vi "NM GlobalTest.vi"() -> ()   [LabVIEW 2010] (continued)
                            tunnel: w1850 -> [w1856 w1873]
                            tunnel: [w1856 w1871] -> w1849
                            tunnel: "data 13" -> [w1860 w1869]
                            tunnel: w1847 -> [w1859 w1868]
                            tunnel: w1846 -> [w1858 w1867]
                            tunnel: [w1857 w1866] -> w1845
                            frame "ULx", Default {
                              n548 = call-poly <vilib>:"ULx Write.vi"("task in"=w1864, "auto start"=w1858, "data"=w1860, "timeout"=w1859, "error in"=w1863) -> ("task out"=w1861:refnum<k24>, "number of samples written per channel"=w1857:u32, "error out"=w1862:errorcluster)  [unwired: 8 in]
                            }
                            frame "DAQmx" {
                              n549 = call-poly <vilib>:"DAQmx Write.vi"("task/channels in"=w1873, "auto start"=w1867, "data"=w1869, "timeout"=w1868, "error in"=w1872) -> ("task out"=w1871:refnum<k21>, "number of samples written per channel"=w1866:u32, "error out"=w1870:errorcluster)  [unwired: 8 in]
                            }
                          }
                        }
                        frame "nCsSU8" {
                          n550 = case shown="\"ULx\", Default" w1882 {
                            tunnel: [w1890 w1894] -> w1884
                            tunnel: [w1891 w1900] -> w1883
                            tunnel: w1881 -> [w1892 w1901]
                            tunnel: w1880 -> [w1893 w1894]
                            tunnel: [w1885 w1899] -> w1879
                            tunnel: w1878 -> [w1885 w1902]
                            tunnel: "data 14" -> [w1889 w1898]
                            tunnel: w1876 -> [w1888 w1897]
                            tunnel: w1875 -> [w1887 w1896]
                            tunnel: [w1886 w1895] -> w1874
                            frame "ULx", Default {
                              n551 = call-poly <vilib>:"ULx Write.vi"("task in"=w1893, "auto start"=w1887, "data"=w1889, "timeout"=w1888, "error in"=w1892) -> ("task out"=w1890:refnum<k24>, "number of samples written per channel"=w1886:u32, "error out"=w1891:errorcluster)  [unwired: 8 in]
                            }
                            frame "DAQmx" {
                              n552 = call-poly <vilib>:"DAQmx Write.vi"("task/channels in"=w1902, "auto start"=w1896, "data"=w1898, "timeout"=w1897, "error in"=w1901) -> ("task out"=w1899:refnum<k21>, "number of samples written per channel"=w1895:u32, "error out"=w1900:errorcluster)  [unwired: 8 in]
                            }
                          }
                        }
                        frame "nCsSU16" {
                          n553 = case shown="\"ULx\", Default" w1911 {
                            tunnel: [w1919 w1929] -> w1913
                            tunnel: [w1921 w1923] -> w1912
                            tunnel: w1910 -> [w1920 w1930]
                            tunnel: w1909 -> [w1922 w1923]
                            tunnel: [w1914 w1928] -> w1908
                            tunnel: w1907 -> [w1914 w1931]
                            tunnel: "data 15" -> [w1918 w1927]
                            tunnel: w1905 -> [w1917 w1925]
                            tunnel: w1904 -> [w1916 w1926]
                            tunnel: [w1915 w1924] -> w1903
                            frame "ULx", Default {
                              n554 = call-poly <vilib>:"ULx Write.vi"("task in"=w1922, "auto start"=w1916, "data"=w1918, "timeout"=w1917, "error in"=w1920) -> ("task out"=w1921:refnum<k24>, "number of samples written per channel"=w1915:u32, "error out"=w1919:errorcluster)  [unwired: 8 in]
                            }
                            frame "DAQmx" {
                              n555 = call-poly <vilib>:"DAQmx Write.vi"("task/channels in"=w1931, "auto start"=w1926, "data"=w1927, "timeout"=w1925, "error in"=w1930) -> ("task out"=w1928:refnum<k21>, "number of samples written per channel"=w1924:u32, "error out"=w1929:errorcluster)  [unwired: 8 in]
                            }
                          }
                        }
                        frame "nCsSU32" {
                          n556 = case shown="\"ULx\", Default" w1939 {
                            tunnel: [w1948 w1952] -> w1942
                            tunnel: [w1949 w1958] -> w1941
                            tunnel: w1940 -> [w1950 w1957]
                            tunnel: w1938 -> [w1951 w1952]
                            tunnel: [w1943 w1959] -> w1937
                            tunnel: w1936 -> [w1943 w1960]
                            tunnel: "data 16" -> [w1947 w1956]
                            tunnel: w1934 -> [w1946 w1955]
                            tunnel: w1933 -> [w1945 w1954]
                            tunnel: [w1944 w1953] -> w1932
                            frame "ULx", Default {
                              n557 = call-poly <vilib>:"ULx Write.vi"("task in"=w1951, "auto start"=w1945, "data"=w1947, "timeout"=w1946, "error in"=w1950) -> ("task out"=w1948:refnum<k24>, "number of samples written per channel"=w1944:u32, "error out"=w1949:errorcluster)  [unwired: 8 in]
                            }
                            frame "DAQmx" {
                              n558 = call-poly <vilib>:"DAQmx Write.vi"("task/channels in"=w1960, "auto start"=w1954, "data"=w1956, "timeout"=w1955, "error in"=w1957) -> ("task out"=w1959:refnum<k21>, "number of samples written per channel"=w1953:u32, "error out"=w1958:errorcluster)  [unwired: 8 in]
                            }
                          }
                        }
                        frame "nCsSWv" {
                          n559 = case shown="\"ULx\", Default" w1969 {
                            tunnel: [w1977 w1981] -> w1971
                            tunnel: [w1978 w1986] -> w1970
                            tunnel: w1968 -> [w1979 w1987]
                            tunnel: w1967 -> [w1980 w1981]
                            tunnel: w1966 -> [w1972 w1989]
                            tunnel: [w1972 w1988] -> w1965
                            tunnel: "data 17" -> [w1976 w1985]
                            tunnel: w1963 -> [w1975 w1984]
                            tunnel: [w1974 w1982] -> w1962
                            tunnel: w1961 -> [w1973 w1983]
                            frame "ULx", Default {
                              n560 = call-poly <vilib>:"ULx Write.vi"("task in"=w1980, "auto start"=w1973, "data"=w1976, "timeout"=w1975, "error in"=w1979) -> ("task out"=w1977:refnum<k24>, "number of samples written per channel"=w1974:u32, "error out"=w1978:errorcluster)  [unwired: 8 in]
                            }
                            frame "DAQmx" {
                              n561 = call-poly <vilib>:"DAQmx Write.vi"("task/channels in"=w1989, "auto start"=w1983, "data"=w1985, "timeout"=w1984, "error in"=w1987) -> ("task out"=w1988:refnum<k21>, "number of samples written per channel"=w1982:u32, "error out"=w1986:errorcluster)  [unwired: 8 in]
                            }
                          }
                        }
                        frame "nCnSU8" {
                          n562 = case shown="\"ULx\", Default" w1998 {
                            tunnel: [w2008 w2010] -> w2000
                            tunnel: [w2007 w2016] -> w1999
                            tunnel: w1997 -> [w2006 w2017]
                            tunnel: w1996 -> [w2009 w2010]
                            tunnel: w1995 -> [w2001 w2018]
                            tunnel: [w2001 w2015] -> w1994
                            tunnel: "data 18" -> [w2005 w2014]
                            tunnel: w1992 -> [w2004 w2013]
                            tunnel: w1991 -> [w2003 w2012]
                            tunnel: [w2002 w2011] -> w1990
                            frame "ULx", Default {
                              n563 = call-poly <vilib>:"ULx Write.vi"("task in"=w2009, "auto start"=w2003, "data"=w2005, "timeout"=w2004, "error in"=w2006) -> ("task out"=w2008:refnum<k24>, "number of samples written per channel"=w2002:u32, "error out"=w2007:errorcluster)  [unwired: 8 in]
                            }
                            frame "DAQmx" {
                              n564 = call-poly <vilib>:"DAQmx Write.vi"("task/channels in"=w2018, "auto start"=w2012, "data"=w2014, "timeout"=w2013, "error in"=w2017) -> ("task out"=w2015:refnum<k21>, "number of samples written per channel"=w2011:u32, "error out"=w2016:errorcluster)  [unwired: 8 in]
                            }
                          }
                        }
                        frame "nCnSU16" {
                          n565 = case shown="\"ULx\", Default" w2027 {
                            tunnel: [w2036 w2044] -> w2029
                            tunnel: [w2035 w2039] -> w2028
                            tunnel: w2026 -> [w2037 w2045]
                            tunnel: w2025 -> [w2038 w2039]
                            tunnel: [w2030 w2046] -> w2024
                            tunnel: w2023 -> [w2030 w2047]
                            tunnel: "data 19" -> [w2034 w2043]
                            tunnel: w2021 -> [w2033 w2042]
                            tunnel: w2020 -> [w2032 w2041]
                            tunnel: [w2031 w2040] -> w2019
                            frame "ULx", Default {
                              n566 = call-poly <vilib>:"ULx Write.vi"("task in"=w2038, "auto start"=w2032, "data"=w2034, "timeout"=w2033, "error in"=w2037) -> ("task out"=w2035:refnum<k24>, "number of samples written per channel"=w2031:u32, "error out"=w2036:errorcluster)  [unwired: 8 in]
                            }
                            frame "DAQmx" {
                              n567 = call-poly <vilib>:"DAQmx Write.vi"("task/channels in"=w2047, "auto start"=w2041, "data"=w2043, "timeout"=w2042, "error in"=w2045) -> ("task out"=w2046:refnum<k21>, "number of samples written per channel"=w2040:u32, "error out"=w2044:errorcluster)  [unwired: 8 in]
                            }
                          }
                        }
                        frame "nCnSU32" {
                          n568 = case shown="\"ULx\", Default" w2056 {
                            tunnel: [w2066 w2068] -> w2058
                            tunnel: [w2065 w2075] -> w2057
                            tunnel: w2055 -> [w2067 w2068]
                            tunnel: w2054 -> [w2064 w2074]
                            tunnel: [w2059 w2076] -> w2053
                            tunnel: w2052 -> [w2059 w2073]
                            tunnel: "data 20" -> [w2063 w2072]
                            tunnel: w2050 -> [w2062 w2071]
                            tunnel: w2049 -> [w2061 w2070]
                            tunnel: [w2060 w2069] -> w2048
                            frame "ULx", Default {
                              n569 = call-poly <vilib>:"ULx Write.vi"("task in"=w2067, "auto start"=w2061, "data"=w2063, "timeout"=w2062, "error in"=w2064) -> ("task out"=w2066:refnum<k24>, "number of samples written per channel"=w2060:u32, "error out"=w2065:errorcluster)  [unwired: 8 in]
                            }
                            frame "DAQmx" {
                              n570 = call-poly <vilib>:"DAQmx Write.vi"("task/channels in"=w2073, "auto start"=w2070, "data"=w2072, "timeout"=w2071, "error in"=w2074) -> ("task out"=w2076:refnum<k21>, "number of samples written per channel"=w2069:u32, "error out"=w2075:errorcluster)  [unwired: 8 in]
                            }
                          }
                        }
                        frame "nCnSWv" {
                          n571 = case shown="\"ULx\", Default" w2085 {
                            tunnel: [w2096 w2105] -> w2087
                            tunnel: [w2095 w2097] -> w2086
                            tunnel: w2084 -> [w2094 w2097]
                            tunnel: w2083 -> [w2088 w2104]
                            tunnel: w2082 -> [w2093 w2103]
                            tunnel: [w2088 w2102] -> w2081
                            tunnel: "data 21" -> [w2092 w2101]
                            tunnel: w2079 -> [w2091 w2100]
                            tunnel: w2078 -> [w2090 w2099]
                            tunnel: [w2089 w2098] -> w2077
                            frame "ULx", Default {
                              n572 = call-poly <vilib>:"ULx Write.vi"("task in"=w2094, "auto start"=w2090, "data"=w2092, "timeout"=w2091, "error in"=w2093) -> ("task out"=w2095:refnum<k24>, "number of samples written per channel"=w2089:u32, "error out"=w2096:errorcluster)  [unwired: 8 in]
                            }
                            frame "DAQmx" {
                              n573 = call-poly <vilib>:"DAQmx Write.vi"("task/channels in"=w2104, "auto start"=w2099, "data"=w2101, "timeout"=w2100, "error in"=w2103) -> ("task out"=w2102:refnum<k21>, "number of samples written per channel"=w2098:u32, "error out"=w2105:errorcluster)  [unwired: 8 in]
                            }
                          }
                        }
                      }
                    }
                    frame "Single Channel" {
                      n574 = call "AtoDSigConvert.vi"("Samples"=w2108, "Array Input"=w2109) -> ("sCnSu32"=w2106:u32[], "sCnSu16"=w2107:u16[], "sCnSu8"=w2110:u8[])
                      n575 = case shown="\"sCnSU32\"" "sDWrite" {
                        tunnel: [w2131 w2161 w2189 w2219 w2247 w2276 w2305 w2335 w2363 w2393] -> w2114
                        tunnel: [w2132 w2160 w2190 w2218 w2248 w2277 w2306 w2334 w2364 w2392] -> w2115
                        tunnel: w2117 -> [w2130 w2158 w2188 w2217 w2245 w2275 w2304 w2333 w2362 w2391]
                        tunnel: w2119 -> [w2128 w2159 w2186 w2215 w2244 w2273 w2302 w2331 w2361 w2390]
                        tunnel: w2120 -> [w2129 w2156 w2184 w2213 w2242 w2272 w2301 w2329 w2358 w2389]
                        tunnel: w2118 -> [w2127 w2157 w2187 w2216 w2246 w2274 w2303 w2332 w2360 w2388]
                        tunnel: [w2126 w2155 w2185 w2214 w2243 w2271 w2300 w2330 w2359 w2387] -> w2116
                        tunnel: w2113 -> [w2123 w2153 w2181 w2210 w2239 w2269 w2298 w2327 w2356 w2384]
                        tunnel: w2112 -> [w2124 w2152 w2182 w2211 w2240 w2267 w2299 w2328 w2357 w2385]
                        tunnel: [w2122 w2151 w2180 w2209 w2238 w2268 w2297 w2326 w2355 w2383] -> w2111
                        tunnel: w2110 -> [_ _ _ _ _ _ w2296 _ _ _]
                        tunnel: w2107 -> [_ _ _ _ _ _ _ w2325 _ _]
                        tunnel: w2106 -> [_ _ _ _ _ _ _ _ w2354 _]
                        frame "sCsSBool", Default {
                          n576 = case shown="\"ULx\", Default" w2130 {
                            tunnel: [w2138 w2142] -> w2132
                            tunnel: [w2139 w2147] -> w2131
                            tunnel: w2129 -> [w2133 w2150]
                            tunnel: w2128 -> [w2141 w2142]
                            tunnel: w2127 -> [w2140 w2148]
                            tunnel: [w2133 w2149] -> w2126
                            tunnel: "data 22" -> [w2137 w2146]
                            tunnel: w2124 -> [w2136 w2145]
                            tunnel: w2123 -> [w2135 w2144]
                            tunnel: [w2134 w2143] -> w2122
                            frame "ULx", Default {
                              n577 = call-poly <vilib>:"ULx Write.vi"("task in"=w2141, "auto start"=w2135, "data"=w2137, "timeout"=w2136, "error in"=w2140) -> ("task out"=w2138:refnum<k24>, "number of samples written per channel"=w2134:u32, "error out"=w2139:errorcluster)  [unwired: 8 in]
                            }
                            frame "DAQmx" {
                              n578 = call-poly <vilib>:"DAQmx Write.vi"("task/channels in"=w2150, "auto start"=w2144, "data"=w2146, "timeout"=w2145, "error in"=w2148) -> ("task out"=w2149:refnum<k21>, "number of samples written per channel"=w2143:u32, "error out"=w2147:errorcluster)  [unwired: 8 in]
                            }
                          }
                        }
                        frame "sCsS1D" {
                          n579 = case shown="\"ULx\", Default" w2158 {
                            tunnel: [w2168 w2176] -> w2161
                            tunnel: [w2167 w2171] -> w2160
                            tunnel: w2159 -> [w2170 w2171]
                            tunnel: w2157 -> [w2169 w2178]
                            tunnel: w2156 -> [w2162 w2179]
                            tunnel: [w2162 w2177] -> w2155
                            tunnel: "data 23" -> [w2166 w2175]
                            tunnel: w2153 -> [w2165 w2173]
                            tunnel: w2152 -> [w2164 w2174]
                            tunnel: [w2163 w2172] -> w2151
                            frame "ULx", Default {
                              n580 = call-poly <vilib>:"ULx Write.vi"("task in"=w2170, "auto start"=w2165, "data"=w2166, "timeout"=w2164, "error in"=w2169) -> ("task out"=w2167:refnum<k24>, "number of samples written per channel"=w2163:u32, "error out"=w2168:errorcluster)  [unwired: 8 in]
                            }
                            frame "DAQmx" {
                              n581 = call-poly <vilib>:"DAQmx Write.vi"("task/channels in"=w2179, "auto start"=w2173, "data"=w2175, "timeout"=w2174, "error in"=w2178) -> ("task out"=w2177:refnum<k21>, "number of samples written per channel"=w2172:u32, "error out"=w2176:errorcluster)  [unwired: 8 in]
                            }
                          }
                        }
                        frame "sCsSU8" {
                          n582 = case shown="\"ULx\", Default" w2188 {
                            tunnel: [w2196 w2200] -> w2190
                            tunnel: [w2197 w2206] -> w2189
                            tunnel: w2187 -> [w2198 w2207]
                            tunnel: w2186 -> [w2199 w2200]
                            tunnel: [w2191 w2205] -> w2185
                            tunnel: w2184 -> [w2191 w2208]
                            tunnel: "data 24" -> [w2195 w2204]
                            tunnel: w2182 -> [w2194 w2203]
                            tunnel: w2181 -> [w2193 w2202]
                            tunnel: [w2192 w2201] -> w2180
                            frame "ULx", Default {
                              n583 = call-poly <vilib>:"ULx Write.vi"("task in"=w2199, "auto start"=w2193, "data"=w2195, "timeout"=w2194, "error in"=w2198) -> ("task out"=w2196:refnum<k24>, "number of samples written per channel"=w2192:u32, "error out"=w2197:errorcluster)  [unwired: 8 in]
                            }
                            frame "DAQmx" {
                              n584 = call-poly <vilib>:"DAQmx Write.vi"("task/channels in"=w2208, "auto start"=w2202, "data"=w2204, "timeout"=w2203, "error in"=w2207) -> ("task out"=w2205:refnum<k21>, "number of samples written per channel"=w2201:u32, "error out"=w2206:errorcluster)  [unwired: 8 in]
                            }
                          }
                        }
                        frame "sCsSU16" {
                          n585 = case shown="\"ULx\", Default" w2217 {
                            tunnel: [w2225 w2235] -> w2219
                            tunnel: [w2227 w2229] -> w2218
                            tunnel: w2216 -> [w2226 w2236]
                            tunnel: w2215 -> [w2228 w2229]
                            tunnel: [w2220 w2234] -> w2214
                            tunnel: w2213 -> [w2220 w2237]
                            tunnel: "data 25" -> [w2224 w2233]
                            tunnel: w2211 -> [w2223 w2232]
                            tunnel: w2210 -> [w2222 w2231]
                            tunnel: [w2221 w2230] -> w2209
                            frame "ULx", Default {
                              n586 = call-poly <vilib>:"ULx Write.vi"("task in"=w2228, "auto start"=w2222, "data"=w2224, "timeout"=w2223, "error in"=w2226) -> ("task out"=w2227:refnum<k24>, "number of samples written per channel"=w2221:u32, "error out"=w2225:errorcluster)  [unwired: 8 in]
                            }
                            frame "DAQmx" {
                              n587 = call-poly <vilib>:"DAQmx Write.vi"("task/channels in"=w2237, "auto start"=w2231, "data"=w2233, "timeout"=w2232, "error in"=w2236) -> ("task out"=w2234:refnum<k21>, "number of samples written per channel"=w2230:u32, "error out"=w2235:errorcluster)  [unwired: 8 in]
                            }
                          }
                        }
                        frame "sCsSU32" {
                          n588 = case shown="\"ULx\", Default" w2245 {
                            tunnel: [w2254 w2258] -> w2248
                            tunnel: [w2255 w2264] -> w2247
                            tunnel: w2246 -> [w2256 w2263]
                            tunnel: w2244 -> [w2257 w2258]
                            tunnel: [w2249 w2265] -> w2243
                            tunnel: w2242 -> [w2249 w2266]
                            tunnel: "data 26" -> [w2253 w2262]
                            tunnel: w2240 -> [w2252 w2261]
                            tunnel: w2239 -> [w2251 w2260]
                            tunnel: [w2250 w2259] -> w2238
                            frame "ULx", Default {
                              n589 = call-poly <vilib>:"ULx Write.vi"("task in"=w2257, "auto start"=w2251, "data"=w2253, "timeout"=w2252, "error in"=w2256) -> ("task out"=w2254:refnum<k24>, "number of samples written per channel"=w2250:u32, "error out"=w2255:errorcluster)  [unwired: 8 in]
                            }
                            frame "DAQmx" {
                              n590 = call-poly <vilib>:"DAQmx Write.vi"("task/channels in"=w2266, "auto start"=w2260, "data"=w2262, "timeout"=w2261, "error in"=w2263) -> ("task out"=w2265:refnum<k21>, "number of samples written per channel"=w2259:u32, "error out"=w2264:errorcluster)  [unwired: 8 in]
                            }
                          }
                        }
                        frame "sCsSWv" {
                          n591 = case shown="\"ULx\", Default" w2275 {
                            tunnel: [w2283 w2287] -> w2277
                            tunnel: [w2284 w2292] -> w2276
                            tunnel: w2274 -> [w2285 w2293]
                            tunnel: w2273 -> [w2286 w2287]
                            tunnel: w2272 -> [w2278 w2295]
                            tunnel: [w2278 w2294] -> w2271
                            tunnel: "data 27" -> [w2282 w2291]
                            tunnel: w2269 -> [w2281 w2289]
                            tunnel: [w2280 w2288] -> w2268
                            tunnel: w2267 -> [w2279 w2290]
                            frame "ULx", Default {
                              n592 = call-poly <vilib>:"ULx Write.vi"("task in"=w2286, "auto start"=w2281, "data"=w2282, "timeout"=w2279, "error in"=w2285) -> ("task out"=w2283:refnum<k24>, "number of samples written per channel"=w2280:u32, "error out"=w2284:errorcluster)  [unwired: 8 in]
                            }
                            frame "DAQmx" {
                              n593 = call-poly <vilib>:"DAQmx Write.vi"("task/channels in"=w2295, "auto start"=w2289, "data"=w2291, "timeout"=w2290, "error in"=w2293) -> ("task out"=w2294:refnum<k21>, "number of samples written per channel"=w2288:u32, "error out"=w2292:errorcluster)  [unwired: 8 in]
                            }
                          }
                        }
                        frame "sCnSU8" {
                          n594 = case shown="\"ULx\", Default" w2304 {
                            tunnel: [w2314 w2316] -> w2306
                            tunnel: [w2313 w2322] -> w2305
                            tunnel: w2303 -> [w2312 w2323]
                            tunnel: w2302 -> [w2315 w2316]
                            tunnel: w2301 -> [w2307 w2324]
                            tunnel: [w2307 w2321] -> w2300
                            tunnel: w2296 -> [w2311 w2320]
                            tunnel: w2299 -> [w2310 w2319]
                            tunnel: w2298 -> [w2309 w2318]
                            tunnel: [w2308 w2317] -> w2297
                            frame "ULx", Default {
                              n595 = call-poly <vilib>:"ULx Write.vi"("task in"=w2315, "auto start"=w2309, "data"=w2311, "timeout"=w2310, "error in"=w2312) -> ("task out"=w2314:refnum<k24>, "number of samples written per channel"=w2308:u32, "error out"=w2313:errorcluster)  [unwired: 8 in]
                            }
                            frame "DAQmx" {
                              n596 = call-poly <vilib>:"DAQmx Write.vi"("task/channels in"=w2324, "auto start"=w2318, "data"=w2320, "timeout"=w2319, "error in"=w2323) -> ("task out"=w2321:refnum<k21>, "number of samples written per channel"=w2317:u32, "error out"=w2322:errorcluster)  [unwired: 8 in]
                            }
                          }
                          "data 28" <- w2296
                        }
                        frame "sCnSU16" {
                          n597 = case shown="\"ULx\", Default" w2333 {
                            tunnel: [w2342 w2350] -> w2335
                            tunnel: [w2341 w2345] -> w2334
                            tunnel: w2332 -> [w2343 w2351]
                            tunnel: w2331 -> [w2344 w2345]
                            tunnel: [w2336 w2352] -> w2330
                            tunnel: w2329 -> [w2336 w2353]
                            tunnel: w2325 -> [w2340 w2349]
                            tunnel: w2328 -> [w2339 w2348]
                            tunnel: w2327 -> [w2338 w2347]
                            tunnel: [w2337 w2346] -> w2326
                            frame "ULx", Default {
                              n598 = call-poly <vilib>:"ULx Write.vi"("task in"=w2344, "auto start"=w2338, "data"=w2340, "timeout"=w2339, "error in"=w2343) -> ("task out"=w2341:refnum<k24>, "number of samples written per channel"=w2337:u32, "error out"=w2342:errorcluster)  [unwired: 8 in]
                            }
                            frame "DAQmx" {
                              n599 = call-poly <vilib>:"DAQmx Write.vi"("task/channels in"=w2353, "auto start"=w2347, "data"=w2349, "timeout"=w2348, "error in"=w2351) -> ("task out"=w2352:refnum<k21>, "number of samples written per channel"=w2346:u32, "error out"=w2350:errorcluster)  [unwired: 8 in]
                            }
                          }
                          "data 29" <- w2325
                        }
                        frame "sCnSU32" {
                          n600 = case shown="\"ULx\", Default" w2362 {
                            tunnel: [w2372 w2374] -> w2364
                            tunnel: [w2371 w2381] -> w2363
                            tunnel: w2361 -> [w2373 w2374]
                            tunnel: w2360 -> [w2370 w2380]
                            tunnel: [w2365 w2382] -> w2359
                            tunnel: w2358 -> [w2365 w2379]
                            tunnel: w2354 -> [w2369 w2378]
                            tunnel: w2357 -> [w2368 w2377]
                            tunnel: w2356 -> [w2367 w2376]
                            tunnel: [w2366 w2375] -> w2355
                            frame "ULx", Default {
                              n601 = call-poly <vilib>:"ULx Write.vi"("task in"=w2373, "auto start"=w2367, "data"=w2369, "timeout"=w2368, "error in"=w2370) -> ("task out"=w2372:refnum<k24>, "number of samples written per channel"=w2366:u32, "error out"=w2371:errorcluster)  [unwired: 8 in]
                            }
                            frame "DAQmx" {
                              n602 = call-poly <vilib>:"DAQmx Write.vi"("task/channels in"=w2379, "auto start"=w2376, "data"=w2378, "timeout"=w2377, "error in"=w2380) -> ("task out"=w2382:refnum<k21>, "number of samples written per channel"=w2375:u32, "error out"=w2381:errorcluster)  [unwired: 8 in]
                            }
                          }
                          "data 30" <- w2354
                        }
                        frame "sCnSWv" {
                          n603 = case shown="\"ULx\", Default" w2391 {
                            tunnel: [w2402 w2411] -> w2393
                            tunnel: [w2401 w2403] -> w2392
                            tunnel: w2390 -> [w2400 w2403]
                            tunnel: w2389 -> [w2394 w2410]
                            tunnel: w2388 -> [w2399 w2409]
                            tunnel: [w2394 w2408] -> w2387
                            tunnel: "data 31" -> [w2398 w2407]
                            tunnel: w2385 -> [w2397 w2406]
                            tunnel: w2384 -> [w2396 w2405]
                            tunnel: [w2395 w2404] -> w2383
                            frame "ULx", Default {
                              n604 = call-poly <vilib>:"ULx Write.vi"("task in"=w2400, "auto start"=w2396, "data"=w2398, "timeout"=w2397, "error in"=w2399) -> ("task out"=w2401:refnum<k24>, "number of samples written per channel"=w2395:u32, "error out"=w2402:errorcluster)  [unwired: 8 in]
                            }
                            frame "DAQmx" {
                              n605 = call-poly <vilib>:"DAQmx Write.vi"("task/channels in"=w2410, "auto start"=w2405, "data"=w2407, "timeout"=w2406, "error in"=w2409) -> ("task out"=w2408:refnum<k21>, "number of samples written per channel"=w2404:u32, "error out"=w2411:errorcluster)  [unwired: 8 in]
                            }
                          }
                        }
                      }
                    }
                  }
                }
                frame "Counter" {
                  n606 = case shown="\"Single Channel\"" "nOrsCChan" {
                    tunnel: w2422 -> [w2432 w2531]
                    tunnel: w2421 -> [w2431 w2530]
                    tunnel: w2420 -> [w2430 w2529]
                    tunnel: w2419 -> [w2433 w2528]
                    tunnel: [w2428 w2526] -> w2417
                    tunnel: [w2427 w2525] -> w2416
                    tunnel: [w2426 w2524] -> w2415
                    tunnel: w2414 -> [w2425 w2523]
                    tunnel: w2413 -> [w2423 w2522]
                    tunnel: [w2424 w2521] -> w2412
                    frame "Multi-Channel", Default {
                      n607 = case shown="\"Frequency\", Default" "nCtrWrite" {
                        tunnel: w2432 -> [w2444 w2472 w2502]
                        tunnel: w2431 -> [w2443 w2471 w2501]
                        tunnel: w2430 -> [w2442 w2470 w2500]
                        tunnel: w2433 -> [w2441 w2473 w2498]
                        tunnel: [w2439 w2468 w2497] -> w2428
                        tunnel: [w2438 w2467 w2496] -> w2427
                        tunnel: [w2437 w2466 w2495] -> w2426
                        tunnel: w2425 -> [w2436 w2465 w2494]
                        tunnel: [w2435 w2463 w2492] -> w2424
                        tunnel: w2423 -> [w2434 w2464 w2493]
                        frame "Frequency", Default {
                          n608 = case shown="\"ULx\", Default" w2441 {
                            tunnel: [w2450 w2454] -> w2438
                            tunnel: [w2451 w2459] -> w2437
                            tunnel: w2444 -> [w2445 w2462]
                            tunnel: w2443 -> [w2453 w2454]
                            tunnel: w2442 -> [w2452 w2460]
                            tunnel: [w2445 w2461] -> w2439
                            tunnel: "data 32" -> [w2449 w2458]
                            tunnel: w2436 -> [w2448 w2457]
                            tunnel: [w2447 w2455] -> w2435
                            tunnel: w2434 -> [w2446 w2456]
                            frame "ULx", Default {
                              n609 = call-poly <vilib>:"ULx Write.vi"("task in"=w2453, "auto start"=w2448, "data"=w2449, "timeout"=w2446, "error in"=w2452) -> ("task out"=w2450:refnum<k24>, "number of samples written per channel"=w2447:u32, "error out"=w2451:errorcluster)  [unwired: 8 in]
                            }
                            frame "DAQmx" {
                              n610 = call-poly <vilib>:"DAQmx Write.vi"("task/channels in"=w2462, "auto start"=w2457, "data"=w2458, "timeout"=w2456, "error in"=w2460) -> ("task out"=w2461:refnum<k21>, "number of samples written per channel"=w2455:u32, "error out"=w2459:errorcluster)  [unwired: 8 in]
                            }
                          }
                        }
                        frame "Time" {
                          n611 = case shown="\"ULx\", Default" w2473 {
                            tunnel: [w2479 w2483] -> w2467
                            tunnel: [w2480 w2488] -> w2466
                            tunnel: w2472 -> [w2474 w2491]
                            tunnel: w2471 -> [w2482 w2483]
                            tunnel: w2470 -> [w2481 w2489]
                            tunnel: [w2474 w2490] -> w2468
                            tunnel: "data 34" -> [w2478 w2487]
                            tunnel: w2465 -> [w2477 w2486]
                            tunnel: w2464 -> [w2476 w2485]
                            tunnel: [w2475 w2484] -> w2463
                            frame "ULx", Default {
                              n612 = call-poly <vilib>:"ULx Write.vi"("task in"=w2482, "auto start"=w2477, "data"=w2478, "timeout"=w2476, "error in"=w2481) -> ("task out"=w2479:refnum<k24>, "number of samples written per channel"=w2475:u32, "error out"=w2480:errorcluster)  [unwired: 8 in]
                            }
                            frame "DAQmx" {
                              n613 = call-poly <vilib>:"DAQmx Write.vi"("task/channels in"=w2491, "auto start"=w2486, "data"=w2487, "timeout"=w2485, "error in"=w2489) -> ("task out"=w2490:refnum<k21>, "number of samples written per channel"=w2484:u32, "error out"=w2488:errorcluster)  [unwired: 8 in]
                            }
                          }
                        }
                        frame "Ticks" {
                          n614 = case shown="\"ULx\", Default" w2498 {
                            tunnel: [w2508 w2512] -> w2496
                            tunnel: [w2509 w2517] -> w2495
                            tunnel: w2502 -> [w2503 w2520]
                            tunnel: w2501 -> [w2511 w2512]
                            tunnel: w2500 -> [w2510 w2518]
                            tunnel: [w2503 w2519] -> w2497
                            tunnel: "data 33" -> [w2507 w2516]
                            tunnel: w2494 -> [w2506 w2515]
                            tunnel: w2493 -> [w2505 w2514]
                            tunnel: [w2504 w2513] -> w2492
                            frame "ULx", Default {
                              n615 = call-poly <vilib>:"ULx Write.vi"("task in"=w2511, "auto start"=w2506, "data"=w2507, "timeout"=w2505, "error in"=w2510) -> ("task out"=w2508:refnum<k24>, "number of samples written per channel"=w2504:u32, "error out"=w2509:errorcluster)  [unwired: 8 in]
                            }
                            frame "DAQmx" {
                              n616 = call-poly <vilib>:"DAQmx Write.vi"("task/channels in"=w2520, "auto start"=w2515, "data"=w2516, "timeout"=w2514, "error in"=w2518) -> ("task out"=w2519:refnum<k21>, "number of samples written per channel"=w2513:u32, "error out"=w2517:errorcluster)  [unwired: 8 in]
                            }
                          }
                        }
                      }
                    }
                    frame "Single Channel" {
                      n617 = case shown="\"Ticks\"" "sCtrWrite" {
                        tunnel: w2531 -> [w2543 w2575 w2606]
                        tunnel: w2530 -> [w2542 w2574 w2605]
                        tunnel: w2529 -> [w2541 w2573 w2604]
                        tunnel: w2528 -> [w2540 w2572 w2607]
                        tunnel: [w2537 w2569 w2601] -> w2526
                        tunnel: [w2536 w2568 w2600] -> w2525
                        tunnel: [w2535 w2567 w2599] -> w2524
                        tunnel: w2523 -> [w2534 w2566 w2598]
                        tunnel: w2522 -> [w2533 w2565 w2597]
                        tunnel: [w2532 w2564 w2596] -> w2521
                        frame "Frequency", Default {
                          n618 = case shown="\"ULx\", Default" w2540 {
                            tunnel: [w2550 w2554] -> w2536
                            tunnel: [w2551 w2560] -> w2535
                            tunnel: w2543 -> [w2544 w2563]
                            tunnel: w2542 -> [w2553 w2554]
                            tunnel: w2541 -> [w2552 w2561]
                            tunnel: [w2544 w2562] -> w2537
                            tunnel: "frequency" -> [w2549 w2559]
                            tunnel: "duty cycle" -> [w2548 w2558]
                            tunnel: w2534 -> [w2547 w2557]
                            tunnel: w2533 -> [w2546 w2556]
                            tunnel: [w2545 w2555] -> w2532
                            frame "ULx", Default {
                              n619 = call-poly <vilib>:"ULx Write.vi"("task in"=w2553, "auto start"=w2547, "frequency"=w2549, "duty cycle"=w2548, "timeout"=w2546, "error in"=w2552) -> ("task out"=w2550:refnum<k24>, "number of samples written per channel"=w2545:u32, "error out"=w2551:errorcluster)  [unwired: 7 in]
                            }
                            frame "DAQmx" {
                              n620 = call-poly <vilib>:"DAQmx Write.vi"("task/channels in"=w2563, "auto start"=w2557, "frequency"=w2559, "duty cycle"=w2558, "timeout"=w2556, "error in"=w2561) -> ("task out"=w2562:refnum<k21>, "number of samples written per channel"=w2555:u32, "error out"=w2560:errorcluster)  [unwired: 7 in]
                            }
                          }
                        }
                        frame "Time" {
                          n621 = case shown="\"ULx\", Default" w2572 {
                            tunnel: [w2582 w2586] -> w2568
                            tunnel: [w2583 w2592] -> w2567
                            tunnel: w2575 -> [w2576 w2595]
                            tunnel: w2574 -> [w2585 w2586]
                            tunnel: w2573 -> [w2584 w2593]
                            tunnel: [w2576 w2594] -> w2569
                            tunnel: "high time" -> [w2581 w2591]
                            tunnel: "low time" -> [w2580 w2590]
                            tunnel: w2566 -> [w2579 w2589]
                            tunnel: w2565 -> [w2578 w2588]
                            tunnel: [w2577 w2587] -> w2564
                            frame "ULx", Default {
                              n622 = call-poly <vilib>:"ULx Write.vi"("task in"=w2585, "auto start"=w2579, "high time"=w2581, "low time"=w2580, "timeout"=w2578, "error in"=w2584) -> ("task out"=w2582:refnum<k24>, "number of samples written per channel"=w2577:u32, "error out"=w2583:errorcluster)  [unwired: 7 in]
                            }
                            frame "DAQmx" {
                              n623 = call-poly <vilib>:"DAQmx Write.vi"("task/channels in"=w2595, "auto start"=w2589, "high time"=w2591, "low time"=w2590, "timeout"=w2588, "error in"=w2593) -> ("task out"=w2594:refnum<k21>, "number of samples written per channel"=w2587:u32, "error out"=w2592:errorcluster)  [unwired: 7 in]
                            }
                          }
                        }
                        frame "Ticks" {
                          n624 = case shown="\"ULx\", Default" w2607 {
                            tunnel: [w2614 w2618] -> w2600
                            tunnel: [w2615 w2624] -> w2599
                            tunnel: w2606 -> [w2608 w2627]
                            tunnel: w2605 -> [w2617 w2618]
                            tunnel: w2604 -> [w2616 w2625]
                            tunnel: [w2608 w2626] -> w2601
                            tunnel: "high ticks" -> [w2613 w2623]
                            tunnel: "low ticks" -> [w2612 w2622]
                            tunnel: w2598 -> [w2611 w2621]
                            tunnel: [w2610 w2619] -> w2596
                            tunnel: w2597 -> [w2609 w2620]
                            frame "ULx", Default {
                              n625 = call-poly <vilib>:"ULx Write.vi"("task in"=w2617, "auto start"=w2611, "high ticks"=w2613, "low ticks"=w2612, "timeout"=w2609, "error in"=w2616) -> ("task out"=w2614:refnum<k24>, "number of samples written per channel"=w2610:u32, "error out"=w2615:errorcluster)  [unwired: 7 in]
                            }
                            frame "DAQmx" {
                              n626 = call-poly <vilib>:"DAQmx Write.vi"("task/channels in"=w2627, "auto start"=w2621, "high ticks"=w2623, "low ticks"=w2622, "timeout"=w2620, "error in"=w2625) -> ("task out"=w2626:refnum<k21>, "number of samples written per channel"=w2619:u32, "error out"=w2624:errorcluster)  [unwired: 7 in]
                            }
                          }
                        }
                      }
                    }
                  }
                }
                frame "Composite" {
                  n627 = local read "ULx"() -> (w2628:refnum<k21>)
                  n628 = local read "ULx"() -> (w2632:refnum<k21>)
                  n629 = Equal?(x=w2628, y="") -> (x = y?=w2629:bool)
                  n630 = Equal?(x=w2632, y="") -> (x = y?=w2631:bool)
                  n631 = call "MultiChanAtoD.vi"("Array Input"=w2636, "Chans"=w2634, "Samples"=w2637) -> ("u32Array"=w2635:u32[][])  [unwired: 1 in, 5 out]
                  n632 = case shown="\"2D\", Default" "CompWrite" {
                    tunnel: w2649 -> [w2665 w2692]
                    tunnel: w2648 -> [w2664 w2691]
                    tunnel: w2647 -> [w2663 w2690]
                    tunnel: w2646 -> [w2666 w2689]
                    tunnel: [w2662 w2686] -> w2645
                    tunnel: [w2661 w2688] -> w2644
                    tunnel: [w2660 w2687] -> w2643
                    tunnel: w2642 -> [w2659 w2685]
                    tunnel: w2641 -> [w2657 w2684]
                    tunnel: [w2658 w2683] -> w2640
                    tunnel: w2639 -> [w2656 _]
                    tunnel: w2638 -> [_ w2682]
                    tunnel: w2635 -> [w2653 _]
                    tunnel: w2631 -> [w2655 _]
                    tunnel: w2629 -> [w2651 _]
                    frame "2D", Default {
                      n633 = case shown="False" w2651 {
                        tunnel: w2653 -> [w2667 _]
                        tunnel: [w2667 _] -> w2652
                        frame False {
                        }
                        frame True {
                        }
                      }
                      n634 = case shown="False" w2655 {
                        tunnel: w2656 -> [w2668 _]
                        tunnel: [w2668 _] -> w2654
                        frame False {
                        }
                        frame True {
                        }
                      }
                      n635 = case shown="\"ULx\", Default" w2666 {
                        tunnel: [w2675 w2679] -> w2660
                        tunnel: [w2676 w2680] -> w2662
                        tunnel: w2665 -> [w2672 w2681]
                        tunnel: w2664 -> [w2678 w2679]
                        tunnel: w2663 -> [w2677 w2680]
                        tunnel: [w2672 w2681] -> w2661
                        tunnel: w2659 -> [w2674 _]
                        tunnel: [w2673 _] -> w2658
                        tunnel: w2657 -> [w2671 _]
                        tunnel: w2652 -> [w2670 _]
                        tunnel: w2654 -> [w2669 _]
                        frame "ULx", Default {
                          n636 = call-poly <vilib>:"ULx Write.vi"("task in"=w2678, "auto start"=w2674, "analog data"=w2669, "digital data"=w2670, "timeout"=w2671, "error in"=w2677) -> ("task out"=w2675:refnum<k24>, "number of samples written per channel"=w2673:u32, "error out"=w2676:errorcluster)  [unwired: 7 in]
                          "DblArray 2" <- w2669
                          "u32Array" <- w2670
                          "u32Plot" <- w2670
                          "DblPlot" <- w2669
                        }
                        frame "DAQmx" {
                        }
                      }
                    }
                    frame "1D Waveform" {
                      n637 = case shown="\"ULx\", Default" w2689 {
                        tunnel: [w2699 w2703] -> w2687
                        tunnel: [w2700 w2704] -> w2686
                        tunnel: w2692 -> [w2694 w2705]
                        tunnel: w2691 -> [w2702 w2703]
                        tunnel: w2690 -> [w2701 w2704]
                        tunnel: [w2694 w2705] -> w2688
                        tunnel: w2685 -> [w2697 _]
                        tunnel: w2684 -> [w2696 _]
                        tunnel: [w2695 _] -> w2683
                        tunnel: w2682 -> [w2693 _]
                        frame "ULx", Default {
                          n638 = call-poly <vilib>:"ULx Write.vi"("task in"=w2702, "auto start"=w2697, "analog data"=w2693, "digital data"="digital data 2", "timeout"=w2696, "error in"=w2701) -> ("task out"=w2699:refnum<k24>, "number of samples written per channel"=w2695:u32, "error out"=w2700:errorcluster)  [unwired: 7 in]
                          "WfmArray" <- w2693
                        }
                        frame "DAQmx" {
                        }
                      }
                    }
                  }
                }
              }
              "writ" <- w1468
              n639 = case shown="True" "Change" {
                tunnel: w1453 -> [_ w1471]
                frame False {
                }
                frame True {
                  n640 = Add(x=w1471, y=1) -> (x+y=w1476:i32)
                  n641 = Greater?(x=w1476, y=3 ("x")) -> (0:w1473:bool)
                  n642 = case shown="True" w1473 {
                    tunnel: [w1477 0] -> w1474
                    tunnel: w1476 -> [w1477 _]
                    frame False {
                    }
                    frame True {
                    }
                  }
                  n643 = property on="sig type" class="Enum (strict)"("Value"=w1474) -> ()  [unwired: 2 in, 2 out]
                }
              }
            }
          }
          n644 = case shown="True" "Once" {
            frame False {
            }
            frame True {
              n645 = local write "Write"(FALSE ("Write")) -> ()
            }
          }
          n646 = local write "Write"(w1427) -> ()
        }
        frame 8 {
          # "STATUS"
          n647 = stacked-sequence {
            seq-local: [w2719 _] -> [_ w2729]
            seq-local: [w2718 _] -> [_ w2728]
            seq-local: [w2717 _] -> [_ w2727]
            tunnel: w2714 -> [w2719 _]
            tunnel: w2713 -> [w2718 _]
            tunnel: w2712 -> [w2717 _]
            tunnel: w2708 -> [_ w2722]
            tunnel: w2707 -> [w2715 _]
            tunnel: [_ w2726] -> w2711
            tunnel: [_ w2725] -> w2710
            tunnel: [_ w2724] -> w2709
            tunnel: [_ FALSE ("Submit")] -> w2706
            frame #0 {
              n648 = for {
                N: 5 -> [_]
                tunnel: w2715 -> [w2720]
                n649 = Wait Until Next ms Multiple(millisecond multiple=w2720) -> ()  [unwired: 1 out]
                "Status" <- TRUE
              }
            }
            frame #1 {
              n650 = while {
                tunnel: w2728 -> [w2742]
                tunnel: w2727 -> [w2741]
                tunnel: [w2740] -> w2725
                tunnel: [w2734] -> w2724
                tunnel: w2722 -> [w2738]
                tunnel: w2729 -> [w2737]
                tunnel: [w2736] -> w2726
                i -> [w2739]
                stop <- w2744 stop-if-true
                n651 = case shown="\"ULx\", Default" w2738 {
                  tunnel: w2742 -> [w2751 w2752]
                  tunnel: w2741 -> [w2750 w2757]
                  tunnel: [w2749 w2752] -> w2740
                  tunnel: [w2748 w2756] -> w2734
                  tunnel: [w2747 w2755] -> w2731
                  tunnel: w2737 -> [w2746 w2754]
                  tunnel: [w2746 w2753] -> w2736
                  frame "ULx", Default {
                    n652 = call <vilib>:"ULx Is Task Done.vi"("task in"=w2751, "error in"=w2750) -> ("task out"=w2749:refnum<k24>, "task done?"=w2747:bool, "error out"=w2748:errorcluster)  [unwired: 11 in]
                  }
                  frame "DAQmx" {
                    n653 = call <vilib>:"DAQmx Is Task Done.vi"("task/channels in"=w2754, "error in"=w2757) -> ("task out"=w2753:refnum<k21>, "task done?"=w2755:bool, "error out"=w2756:errorcluster)  [unwired: 11 in]
                  }
                }
                "task \ndone?" <- w2731
                n654 = Wait Until Next ms Multiple(millisecond multiple=u32 300) -> ()  [unwired: 1 out]
                n655 = call "TextError.vi"("error in"=w2734) -> ("message"=w2733:string)  [unwired: 1 in]
                n656 = local read "Status\nLoop"() -> (w2732:bool)
                n657 = local write "message 2"(w2733) -> ()
                n658 = Not(x=w2732) -> (.not. x?=w2730:bool)
                n659 = local read "Submit"() -> (w2745:bool)
                n660 = local read "stop"() -> (w2743:bool)
                n661 = Compound Arithmetic op=OR(w2731, w2730, w2743, w2745) -> (w2744:bool)
                "# of Loops" <- w2739
              }
            }
          }
          n662 = local write "Status"(w2706) -> ()
          n663 = local write "Submit"(w2706) -> ()
        }
        frame 9 {
          # "STOP"
          n664 = for {
            N: 5 -> [_]
            tunnel: w2760 -> [w2772]
            tunnel: [FALSE] -> w2759
            n665 = Wait Until Next ms Multiple(millisecond multiple=w2772) -> ()  [unwired: 1 out]
            "Stop" <- TRUE
          }
          n666 = case shown="\"ULx\", Default" w2768 {
            tunnel: [w2778 w2779] -> w2763
            tunnel: w2766 -> [w2777 w2779]
            tunnel: w2765 -> [w2776 w2782]
            tunnel: [w2775 w2783] -> w2762
            tunnel: w2767 -> [w2774 w2781]
            tunnel: [w2774 w2780] -> w2764
            frame "ULx", Default {
              n667 = call <vilib>:"ULx Stop Task.vi"("error in"=w2776, "task in"=w2777) -> ("error out"=w2775:errorcluster, "task out"=w2778:refnum<k24>)  [unwired: 8 in]
            }
            frame "DAQmx" {
              n668 = call <vilib>:"DAQmx Stop Task.vi"("task/channels in"=w2781, "error in"=w2782) -> ("task out"=w2780:refnum<k21>, "error out"=w2783:errorcluster)  [unwired: 12 in]
            }
          }
          n669 = local write "Stop"(w2759) -> ()
          n670 = case shown="True" "Once" {
            frame False {
            }
            frame True {
              n671 = local write "Stop"(FALSE ("Stop")) -> ()
            }
          }
          "Task Stopped" <- TRUE
        }
        frame 10 {
          # "CLEAR"
          n672 = for {
            N: 5 -> [_]
            tunnel: w2785 -> [w2796]
            tunnel: [FALSE] -> w2784
            n673 = Wait Until Next ms Multiple(millisecond multiple=w2796) -> ()  [unwired: 1 out]
            "Clear" <- TRUE
          }
          n674 = local write "Clear"(w2784) -> ()
          n675 = case shown="\"ULx\", Default" w2791 {
            tunnel: w2793 -> [w2801 w2802]
            tunnel: w2792 -> [w2800 w2804]
            tunnel: [w2799 w2805] -> w2787
            tunnel: w2794 -> [w2798 w2803]
            tunnel: [w2798 _] -> w2789
            tunnel: [_ w2802] -> w2788
            frame "ULx", Default {
              n676 = call <vilib>:"ULx Clear Task.vi"("task in"=w2801, "error in"=w2800) -> ("error out"=w2799:errorcluster)  [unwired: 13 in]
            }
            frame "DAQmx" {
              n677 = call <vilib>:"DAQmx Clear Task.vi"("task in"=w2803, "error in"=w2804) -> ("error out"=w2805:errorcluster)  [unwired: 13 in]
            }
          }
          "Task Cleared" <- TRUE
        }
        frame 11 {
          # "READ"
          n678 = stacked-sequence {
            tunnel: w2815 -> [_ w2829]
            tunnel: w2814 -> [_ w2828]
            tunnel: w2813 -> [_ w2827]
            tunnel: w2812 -> [_ w2826]
            tunnel: [_ w2825] -> w2811
            tunnel: [_ w2824] -> w2810
            tunnel: [_ w2823] -> w2809
            tunnel: w2808 -> [w2817 _]
            tunnel: [_ FALSE] -> w2807
            frame #0 {
              n679 = for {
                N: 5 -> [_]
                tunnel: w2817 -> [w2820]
                n680 = Wait Until Next ms Multiple(millisecond multiple=w2820) -> ()  [unwired: 1 out]
                "Read" <- TRUE ("Write")
              }
            }
            frame #1 {
              n681 = case shown="\"Digital\"" "ReadType" {
                tunnel: w2828 -> [w2838 w3126 w3637 w3842]
                tunnel: w2827 -> [w2837 w3125 w3638 w3843]
                tunnel: w2829 -> [w2836 w3127 w3636 w3841]
                tunnel: w2826 -> [w2835 w3121 w3632 w3837]
                tunnel: [w2834 w3122 w3635 w3840] -> w2825
                tunnel: [w2833 w3123 w3634 w3839] -> w2824
                tunnel: [w2832 w3124 w3633 w3838] -> w2823
                tunnel: "timeout" -> [w2831 w3120 w3631 w3835]
                frame "Analog", Default {
                  n682 = case shown="\"sCnS1D\"" "ARead" {
                    tunnel: [w2847 w2871 w2894 w2921 w2945 w2968 w2992 w3019 w3041 w3062 w3083 w3104] -> w2832
                    tunnel: [w2848 w2870 w2895 w2920 w2946 w2969 w2993 w3018 w3039 w3059 w3080 w3101] -> w2833
                    tunnel: w2838 -> [w2845 w2869 w2889 w2918 w2943 w2966 w2990 w3016 w3044 w3064 w3085 w3106]
                    tunnel: w2836 -> [w2846 w2867 w2891 w2916 w2941 w2965 w2989 w3014 w3045 w3063 w3084 w3105]
                    tunnel: w2837 -> [w2844 w2868 w2893 w2919 w2944 w2967 w2991 w3017 w3043 w3065 w3086 w3107]
                    tunnel: [w2843 w2866 w2892 w2917 w2942 w2964 w2988 w3015 w3042 w3061 w3082 w3103] -> w2834
                    tunnel: w2835 -> [w2841 w2864 w2888 w2914 w2939 w2962 w2986 w3012 w3038 w3058 w3079 w3100]
                    tunnel: w2831 -> [w2840 w2863 w2887 w2913 w2938 w2961 w2985 w3011 w3036 w3057 w3078 w3099]
                    frame "sCsSDbl", Default {
                      n683 = case shown="\"DAQmx\"" w2841 {
                        tunnel: [w2854 w2857] -> w2848
                        tunnel: [w2853 w2860] -> w2847
                        tunnel: [w2855 w2862] -> w2842
                        tunnel: w2846 -> [w2850 w2859]
                        tunnel: w2845 -> [w2852 w2857]
                        tunnel: w2844 -> [w2851 w2858]
                        tunnel: [w2850 w2861] -> w2843
                        tunnel: w2840 -> [w2849 w2856]
                        frame "ULx", Default {
                          n684 = call-poly <vilib>:"ULx Read.vi"("task in"=w2852, "timeout"=w2849, "error in"=w2851) -> ("task out"=w2854:refnum<k24>, "data"=w2855:dbl, "error out"=w2853:errorcluster)  [unwired: 10 in]
                        }
                        frame "DAQmx" {
                          n685 = call-poly <vilib>:"DAQmx Read.vi"("task/channels in"=w2859, "timeout"=w2856, "error in"=w2858) -> ("task out"=w2861:refnum<k21>, "data"=w2862:dbl, "error out"=w2860:errorcluster)  [unwired: 10 in]
                        }
                      }
                      "data 35" <- w2842
                    }
                    frame "sCsSWfm" {
                      n686 = case shown="\"DAQmx\"" w2864 {
                        tunnel: [w2876 w2883] -> w2871
                        tunnel: [w2877 w2880] -> w2870
                        tunnel: [w2878 w2885] -> w2865
                        tunnel: w2869 -> [w2874 w2880]
                        tunnel: w2868 -> [w2875 w2882]
                        tunnel: w2867 -> [w2873 w2881]
                        tunnel: [w2873 w2884] -> w2866
                        tunnel: w2863 -> [w2872 w2879]
                        frame "ULx", Default {
                          n687 = call-poly <vilib>:"ULx Read.vi"("task in"=w2874, "timeout"=w2872, "error in"=w2875) -> ("task out"=w2877:refnum<k24>, "data"=w2878:waveform(dbl), "error out"=w2876:errorcluster)  [unwired: 10 in]
                        }
                        frame "DAQmx" {
                          n688 = call-poly <vilib>:"DAQmx Read.vi"("task/channels in"=w2881, "timeout"=w2879, "error in"=w2882) -> ("task out"=w2884:refnum<k21>, "data"=w2885:waveform(dbl), "error out"=w2883:errorcluster)  [unwired: 10 in]
                        }
                      }
                      "data 36" <- w2865
                    }
                    frame "sCnS1D" {
                      n689 = case shown="\"DAQmx\"" w2888 {
                        tunnel: [w2902 w2907] -> w2895
                        tunnel: [w2901 w2910] -> w2894
                        tunnel: [w2903 w2906] -> w2890
                        tunnel: w2893 -> [w2899 w2909]
                        tunnel: w2889 -> [w2900 w2907]
                        tunnel: [w2898 w2911] -> w2892
                        tunnel: w2891 -> [w2898 w2908]
                        tunnel: w2887 -> [w2897 w2905]
                        tunnel: "samples per" -> [w2896 w2904]
                        frame "ULx", Default {
                          n690 = call-poly <vilib>:"ULx Read.vi"("task in"=w2900, "number of samples per channel"=w2896, "timeout"=w2897, "error in"=w2899) -> ("task out"=w2902:refnum<k24>, "data"=w2903:dbl[], "error out"=w2901:errorcluster)  [unwired: 9 in]
